vi "DrawWhiteKey.vi"(6 "KeyNumber":i32=52, 7 "WhiteKeySize":cluster{"Width":i32, "Hieght":i32}={"Width"=21, "Hieght"=147}, 8 "error in (no error)":errorcluster, 10 "WhiteKeyData array":u32[][](array[numeric]), 11 "Image In":T1) -> (0 "error out":errorcluster, 3 "Image Out":T1)   [LabVIEW 2015]
uses:
  <vilib>/vision/Image Controls.llb/IMAQ Image.ctl
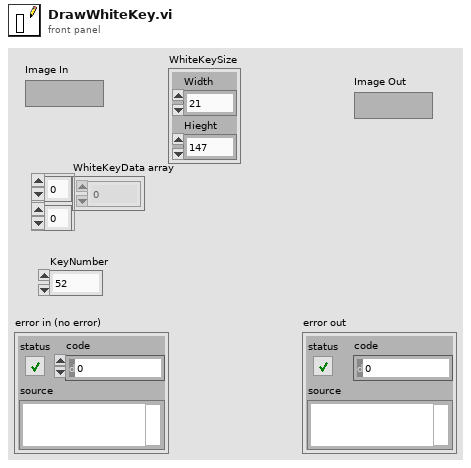
[diagram p1: front panel]
types:
  T1 = typedef "IMAQ Image.ctl" = refnum<image>
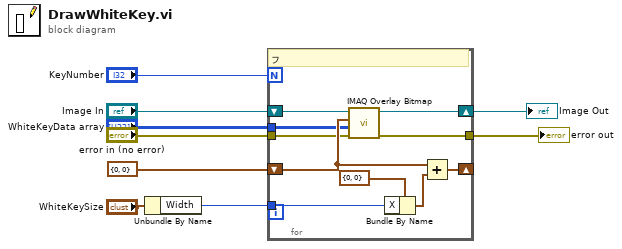
[diagram p0: block diagram]
diagram:
  n1 = Unbundle By Name("WhiteKeySize") -> ("Width"=w2:i32)
  n2 = for {
    N: "KeyNumber" -> [_]
    shift-right: [w18] -> w5
    shift-left: "Image In" -> [w19]
    shift-right: [w16] -> _
    shift-left: cluster{"X":i32, "Y":i32} {"X"=0, "Y"=0} ("Top Left Point") -> [w17]
    tunnel: w2 -> [w12]
    tunnel: "error in (no error)" -> [w13]
    tunnel: [w11] -> w6
    tunnel: "WhiteKeyData array" -> [w10]
    # "フ"
    n3 = call "IMAQ Overlay Bitmap"("error in (no error)"=w13, "Bitmap"=w10, "Top Left Point"=w17, "Image"=w19) -> ("error out"=w11:errorcluster, "Image Out"=w18:T1)  [unwired: 6 in]
    n4 = Bundle By Name(cluster=cluster{"X":i32, "Y":i32} {"X"=0, "Y"=0} ("y"), "X"=w12) -> (w14:cluster{"X":i32, "Y":i32})
    n5 = Add(x=w17, y=w14) -> (x+y=w16:cluster{"X":i32, "Y":i32})
  }
  "Image Out" <- w5
  "error out" <- w6
